vi "PlotCylparams_ILThack.vi"() -> ()   [LabVIEW 2014]
uses:
  TypeDefs/RectHatch.ctl
  TypeDefs/PowerSpeed.ctl
  <vilib>/Utility/file.llb/Read From Spreadsheet File (DBL).vi
panel:
  out "Params":cluster{dbl, dbl, dbl, dbl, dbl}[](array[cluster])
  in  "CircHatch":T1={"Diameter"=1.6, "Angle"=45.0, "Offset"=0.05, "Spacing"=0.1} {"Spacing" format="%#_13g"; "Offset" format="%#_13g"; "Diameter" format="%#_13g"}
  in  "DummyCubeLoc":cluster{dbl, dbl}={-30.0, 30.0}
  in  "Save?":bool=TRUE
  in  "Path":path=path "\\\\nif-prgms-srvr.llnl.gov\\LMOT/Damage Group/Matthews/AM/fraunhofer SLM/BuildFiles_STL_ILT/SCN/DogBoneAndCylinders_11-23-16"
  in  "HighPower":dbl=300.0
  in  "Display":T2={"Mode"=enum."Inherit Value", "PointSize"=1.0, "LineWidth"=1.0}
  in  "LayerEnd":u32=266
  in  "LayerStart":u32
  in  "HatchPow":T3={"Power"=350.0, "Mark Speed"=300.0, "Jump Speed"=1000.0}
  in  "RectHatch":T4={"Width"=10.0, "Height"=1.0, "Angle"=45.0, "OffX"=0.1, "OffY"=0.1, "Spacing"=0.1} {"Spacing" format="%#_13g"; "OffY" format="%#_13g"; "OffX" format="%#_13g"; "Height" format="%#_13g"; "Width" format="%#_13g"}
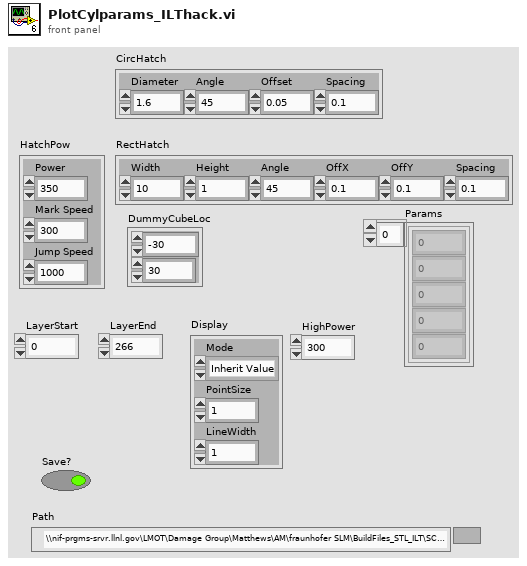
[diagram p1: front panel]
types:
  T1 = cluster{"Diameter":dbl, "Angle":sgl, "Offset":dbl, "Spacing":dbl}
  T2 = cluster{"Mode":enum16{"Inherit Value", "Points", "Wireframe", "Polygons"}, "PointSize":sgl, "LineWidth":sgl}
  T3 = typedef "PowerSpeed.ctl" = cluster{"Power":dbl, "Mark Speed":dbl, "Jump Speed":dbl}
  T4 = typedef "RectHatch.ctl" = cluster{"Width":dbl, "Height":dbl, "Angle":sgl, "OffX":dbl, "OffY":dbl, "Spacing":dbl}
  T5 = typedef "PathSupreme.ctl" = cluster{"VelocityProfiles":T6[], "Path":T7}
  T6 = typedef "VelocityProfile.ctl" = cluster{"ID":u32, "Velocity":dbl, "Mode":string, "tV1":u32, "tV2":u32, "tL1":u32, "tL2":u32}
  T7 = typedef "PathCut.ctl" = cluster{"Type":string, "Tag":string, "Segments":T8[]}
  T8 = typedef "Segment.ctl" = cluster{"SegmentID":u16, "Power":sgl, "idxVelocityProfile":u16, "End":cluster{"X":sgl, "Y":sgl}}
  T9 = cluster{"Start":cluster{"X":dbl, "Y":dbl}, "End":cluster{"X":dbl, "Y":dbl}}[]
  T10 = typedef "Point3D.ctl" = cluster{"X":sgl, "Y":sgl, "Z":sgl}
  T11 = cluster{"Hatches":cluster{"Start":cluster{"X":dbl, "Y":dbl}, "End":cluster{"X":dbl, "Y":dbl}}[]}
  T12 = cluster{"Hatches":cluster{"Start":cluster{"X":dbl, "Y":dbl}, "End":cluster{"X":dbl, "Y":dbl}}[]}[]
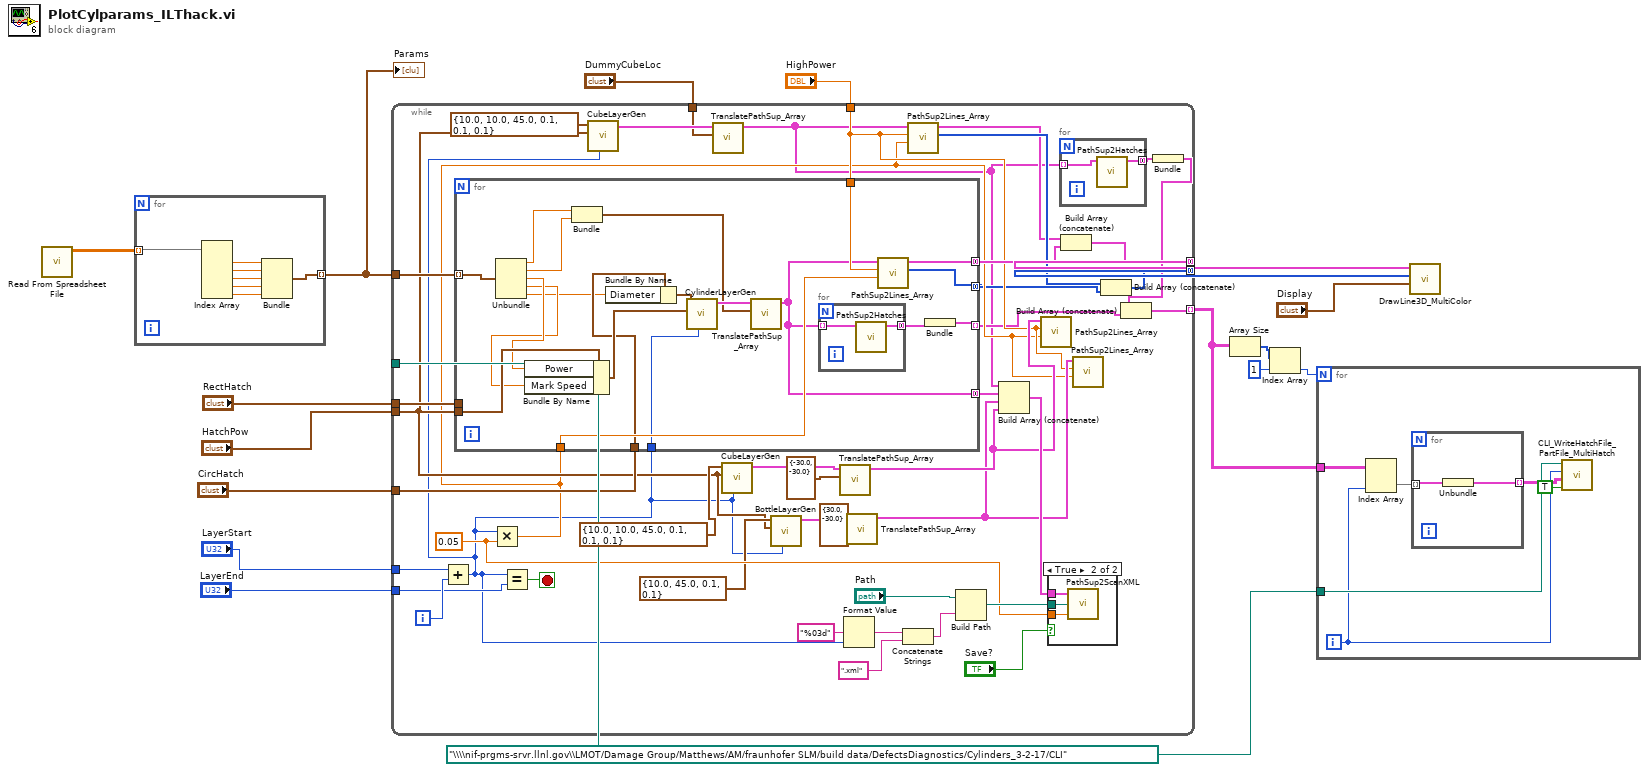
[diagram p0: block diagram]
diagram:
  w1 = path "\\\\nif-prgms-srvr.llnl.gov\\LMOT/Damage Group/Matthews/AM/fraunhofer SLM/build data/DefectsDiagnostics/Cylinders_3-2-17/CLI" ("Path")
  n1 = call-poly <vilib>:"Read From Spreadsheet File.vi"() -> ("all rows"=w17:dbl[][])  [unwired: 7 in, 4 out]
  n2 = for {
    tunnel: w17 -> [w24] mode=indexing
    tunnel: [w19] -> w12 mode=indexing
    n3 = Index Array(array=w24) -> (element #1=w22:dbl, element #2=w23:dbl, element #3=w21:dbl, element #4=w20:dbl, element #5=w18:dbl)  [unwired: 5 in]
    n4 = Bundle(w22, w23, w21, w20, w18) -> (w19:cluster{dbl, dbl, dbl, dbl, dbl})  [unwired: 1 in]
  }
  "Params" <- w12
  n5 = while {
    tunnel: "HighPower" -> [w35]
    tunnel: [w51] -> w15 mode=concatenating
    tunnel: [w50] -> w14 mode=concatenating
    tunnel: w12 -> [w65]
    tunnel: "RectHatch" -> [w47]
    tunnel: "HatchPow" -> [w40]
    tunnel: "LayerEnd" -> [w64]
    tunnel: "LayerStart" -> [w63]
    tunnel: "DummyCubeLoc" -> [w53]
    tunnel: "CircHatch" -> [w46]
    tunnel: w1 -> [_]
    tunnel: [w27] -> w2 mode=indexing
    i -> [w67]
    stop <- w66 stop-if-true
    w56 = 0.05 ("y")
    n6 = Add(x=w63, y=w67) -> (x+y=w33:u32)
    n7 = Multiply(x=w33, y=w56) -> (x*y=w34:dbl)
    n8 = for {
      tunnel: w33 -> [w76]
      tunnel: w34 -> [w90]
      tunnel: w35 -> [w89]
      tunnel: [w92] -> w52 mode=concatenating
      tunnel: w65 -> [w91] mode=indexing
      tunnel: w47 -> [_]
      tunnel: w40 -> [w87]
      tunnel: [w75] -> w49 mode=concatenating
      tunnel: [w88] -> w32 mode=concatenating
      tunnel: w46 -> [w79]
      tunnel: [w73] -> w30 mode=indexing
      n9 = Unbundle(w91) -> (w80:dbl, w83:dbl, w86:dbl, w85:dbl, w77:dbl)
      n10 = Bundle By Name(cluster=w87, "Power"=w86, "Mark Speed"=w85) -> (w84:T3)
      n11 = Bundle(w80, w83) -> (w81:cluster{dbl, dbl})  [unwired: 1 in]
      n12 = Bundle By Name(cluster=w79, "Diameter"=w77) -> (w78:T1)
      n13 = call "CylinderLayerGen.vi"("Layer"=w76, "HatchPow"=w84, "CircHatch"=w78) -> ("PathSups"=w82:T5[])  [unwired: 8 in]
      n14 = call "TranslatePathSup_Array.vi"("Offset"=w81, "PathSupsIn"=w82) -> ("PathSupsOut"=w75:T5[])  [unwired: 9 in]
      n15 = for {
        tunnel: w75 -> [w94] mode=indexing
        tunnel: [w93] -> w74 mode=concatenating
        n16 = call "PathSup2Hatches.vi"("PathSupOut"=w94) -> ("Hatches"=w93:T9)  [unwired: 10 in]
      }
      n17 = call "PathSup2Lines_Array.vi"("Z"=w90, "HighPower"=w89, "PathSupIn"=w75) -> ("Colors"=w88:u32[], "Lines"=w92:cluster{"P0":T10, "P1":T10}[])  [unwired: 7 in]
      n18 = Bundle("Hatches"=w74) -> (w73:T11)  [unwired: 1 in]
    }
    n19 = Equal?(x=w33, y=w64) -> (x = y?=w66:bool)
    n20 = call "CubeLayerGen.vi"("Layer"=w33, "HatchPow"=w40, "RectHatch"=T4 {"Width"=10.0, "Height"=10.0, "Angle"=45.0, "OffX"=0.1, "OffY"=0.1, "Spacing"=0.1}) -> ("PathSups"=w54:T5[])  [unwired: 8 in]
    n21 = call "TranslatePathSup_Array.vi"("Offset"=w53, "PathSupsIn"=w54) -> ("PathSupsOut"=w28:T5[])  [unwired: 9 in]
    n22 = call "CubeLayerGen.vi"("Layer"=w33, "HatchPow"=w40, "RectHatch"=T4 {"Width"=10.0, "Height"=10.0, "Angle"=45.0, "OffX"=0.1, "OffY"=0.1, "Spacing"=0.1}) -> ("PathSups"=w43:T5[])  [unwired: 8 in]
    n23 = call "BottleLayerGen.vi"("Layer"=w33, "HatchPow"=w40, "CircHatch"=T1 {"Diameter"=10.0, "Angle"=45.0, "Offset"=0.1, "Spacing"=0.1}) -> ("PathSups"=w39:T5[])  [unwired: 8 in]
    n24 = call "TranslatePathSup_Array.vi"("Offset"=cluster{dbl, dbl} {-30.0, -30.0}, "PathSupsIn"=w43) -> ("PathSupsOut"=w37:T5[])  [unwired: 9 in]
    n25 = Format Value(format string="%03d", value (0)=w33) -> (output string=w61:string)  [unwired: 1 in]
    n26 = call "TranslatePathSup_Array.vi"("Offset"=cluster{dbl, dbl} {30.0, -30.0}, "PathSupsIn"=w39) -> ("PathSupsOut"=w36:T5[])  [unwired: 9 in]
    n27 = Concatenate Strings(w61, ".xml" ("string")) -> (w59:string)
    n28 = call "PathSup2Lines_Array.vi"("Z"=w34, "HighPower"=w35, "PathSupIn"=w28) -> ("Colors"=w31:u32[], "Lines"=w29:cluster{"P0":T10, "P1":T10}[])  [unwired: 7 in]
    n29 = Build Path(base path="Path", name or relative path=w59) -> (appended path=w57:path)
    n30 = Build Array (concatenate)(w28, w49, w36, w37) -> (w48:T5[])
    n31 = call "PathSup2Lines_Array.vi"("Z"=w34, "HighPower"=w35, "PathSupIn"=w37) -> ()  [unwired: 7 in, 2 out]
    n32 = case shown="True" "Save?" {
      tunnel: w48 -> [_ w72]
      tunnel: w57 -> [_ w71]
      tunnel: w56 -> [_ w70]
      frame False {
      }
      frame True {
        n33 = call "PathSup2ScanXML.vi"("Thickness"=w70, "Path"=w71, "PathSupremes"=w72) -> ()  [unwired: 2 in, 1 out]
      }
    }
    n34 = for {
      tunnel: [w69] -> w26 mode=concatenating
      tunnel: w28 -> [w68] mode=indexing
      n35 = call "PathSup2Hatches.vi"("PathSupOut"=w68) -> ("Hatches"=w69:T9)  [unwired: 10 in]
    }
    n36 = Build Array (concatenate)(w29, w52) -> (w51:cluster{"P0":T10, "P1":T10}[])
    n37 = call "PathSup2Lines_Array.vi"("Z"=w34, "HighPower"=w35, "PathSupIn"=w36) -> ()  [unwired: 7 in, 2 out]
    n38 = Build Array (concatenate)(w31, w32) -> (w50:u32[])
    n39 = Bundle("Hatches"=w26) -> (w25:T11)  [unwired: 1 in]
    n40 = Build Array (concatenate)(w25, w30) -> (w27:T12)
  }
  n41 = Array Size(array=w2) -> (size(s)=w5:i32[])
  n42 = Index Array(array=w5, index=1) -> (element=w4:i32)
  n43 = for {
    N: w4 -> [_]
    tunnel: w2 -> [w100]
    tunnel: w1 -> [w97]
    i -> [w96]
    n44 = Index Array(array=w100, index (col)=w96) -> (element=w99:T12)  [unwired: 1 in]
    n45 = for {
      tunnel: w99 -> [w102] mode=indexing
      tunnel: [w101] -> w98 mode=indexing
      n46 = Unbundle(w102) -> ("Hatches"=w101:T9)
    }
    n47 = call "CLI_WriteHatchFile_PartFile_MultiHatch.vi"("Write?"=TRUE, "Hatches"=w98, "PartNum"=w96, "Path"=w97) -> ()  [unwired: 7 in, 1 out]
  }
  n48 = call "DrawLine3D_MultiColor.vi"("Display"="Display", "Colors"=w14, "Lines"=w15) -> ()  [unwired: 9 in]
